vi "ChangeSetpoint.vi"(8 "error in (no error)":errorcluster, 9 "数组":dbl[](array[numeric]), 10 "Setpoint":dbl, 11 "SignalSenderLoop":refnum<class "SignalSenderLoop.lvclass">) -> (0 "error out":errorcluster, 3 "SignalSenderLoop out":refnum<class "SignalSenderLoop.lvclass">)   [LabVIEW 2020, in "ECU_Diagnose.lvlib" / "SignalSenderLoop.lvclass"]
doc: "---------------------------------------------------------------\nJKI State Machine Objects™\nhttp://jki.net/state-machine-objects/\nCopyright (C) 2005-2015, JKI <info@jki.net>\nALL RIGHTS RESERVEDJKI State Machine Objects (SMO) 1.0.0.5\nJKI - JKI\nCopyright (c) 2016, JKI"
uses:
  SignalSenderLoop.lvclass
panel:
  # "For instructions on how to use the JKI State Machine Objects, examples and video tutorials, visit:\nhttp://jki.net/state-machine-objects/\n\nJKI State Machine Objects™\nhttp://jki.net/state-machine-objects/\nCopyright (C) 2005-2015, JKI <info@jki.net>\nALL RIGHTS RESERVED"
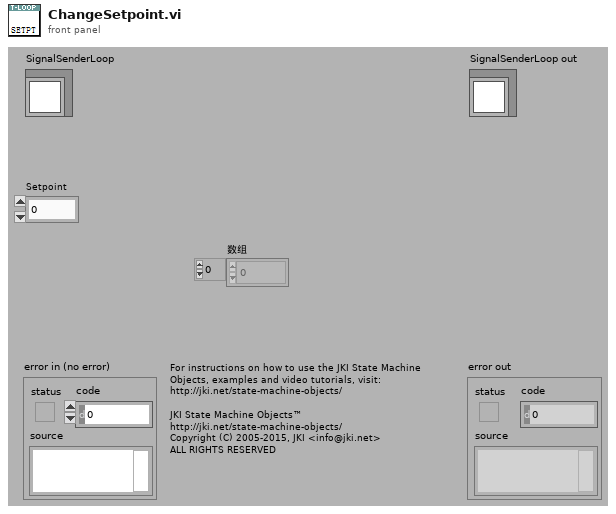
[diagram p1: front panel]
types:
  T1 = typedef "ECU_Diagnose.lvlib/SignalSenderLoop.lvclass/PrivateEvents--Cluster.ctl" = cluster{"AsyncMethod":refnum<user-event>, "SignalCMDArry":refnum<user-event>}
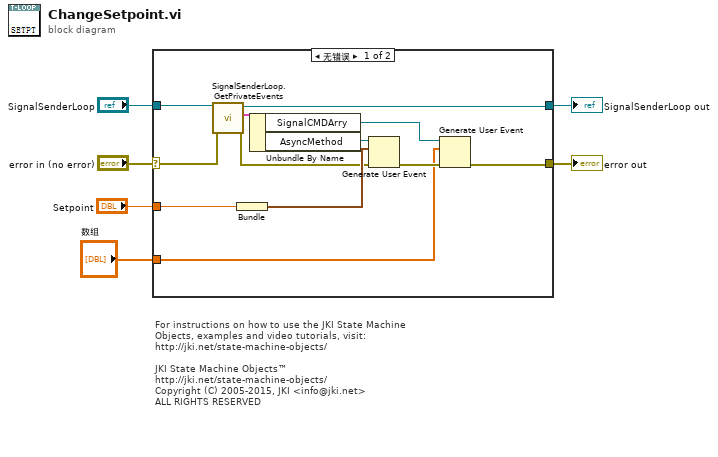
[diagram p0: block diagram]
diagram:
  # "For instructions on how to use the JKI State Machine Objects, examples and video tutorials, visit:\nhttp://jki.net/state-machine-objects/\n\nJKI State Machine Objects™\nhttp://jki.net/state-machine-objects/\nCopyright (C) 2005-2015, JKI <info@jki.net>\nALL RIGHTS RESERVED"
  n1 = case shown="无错误" "error in (no error)" {
    selector: "error in (no error)" -> [w17 w19]
    tunnel: "SignalSenderLoop" -> [w18 w20]
    tunnel: [w9 w19] -> w5
    tunnel: [w16 w20] -> w4
    tunnel: "Setpoint" -> [w13 _]
    tunnel: "数组" -> [w7 _]
    frame No Error {
      n2 = call "SignalSenderLoop.GetPrivateEvents.vi"("error in (no error)"=w17, "SignalSenderLoop"=w18) -> ("error out"=w11:errorcluster, "Private Events"=w15:T1, "SignalSenderLoop out"=w16:refnum<class "SignalSenderLoop.lvclass">)  [unwired: 7 in]
      n3 = Bundle("Setpoint"=w13) -> (w12:cluster{"Setpoint":dbl})  [unwired: 1 in]
      n4 = Unbundle By Name(w15) -> ("SignalCMDArry"=w8:refnum<user-event>, "AsyncMethod"=w14:refnum<user-event>)
      n5 = Generate User Event(user event=w14, event data cluster=w12, error in=w11) -> (error out=w10:errorcluster)  [unwired: 1 in, 1 out]
      n6 = Generate User Event(user event=w8, event data cluster=w7, error in=w10) -> (error out=w9:errorcluster)  [unwired: 1 in, 1 out]
    }
    frame Error {
    }
  }
  "error out" <- w5
  "SignalSenderLoop out" <- w4
